vi "MdfSave.vi"(8 "error in (no error)":errorcluster, 10 "stop_time":u64, 11 "MDFRef":refnum<k24>) -> (0 "error IO":errorcluster, 2 "FinalizeMeasurement":bool, 3 "MDFRef out":refnum<k24>)   [LabVIEW 2025, in "MdfFile.lvlib"]
uses:
  MdfFile.lvlib
  data/mdflibrary.dll
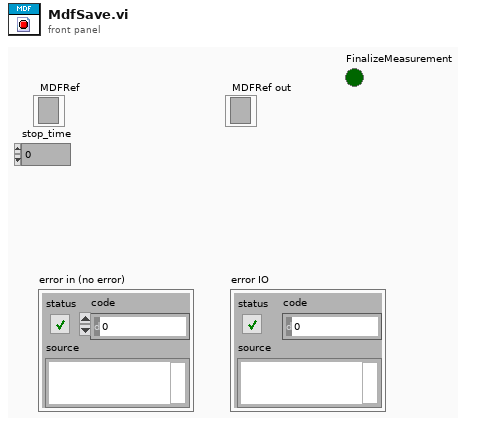
[diagram p1: front panel]
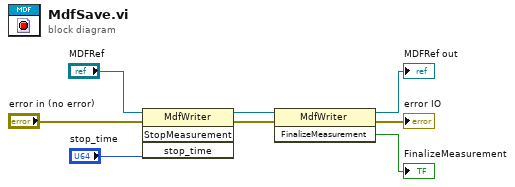
[diagram p0: block diagram]
diagram:
  n1 = invoke class="MdfWriter" method="StopMeasurement"(reference="MDFRef", error in="error in (no error)", "stop_time"="stop_time") -> (reference out=w5:refnum<k24>, error out=w3:errorcluster)  [unwired: 1 in, 2 out]
  n2 = invoke class="MdfWriter" method="FinalizeMeasurement"(reference=w5, error in=w3) -> (reference out=→"MDFRef out":refnum<k24>, error out=→"error IO":errorcluster, "FinalizeMeasurement"=→"FinalizeMeasurement":bool)  [unwired: 1 in]
